vi "arduino -- check responce.vi"(11 "resonse":string) -> (2 "ok?":bool)   [LabVIEW 2020]
uses:
  <vilib>/regexp/Match Regular Expression.xnode
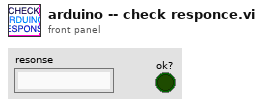
[diagram p1: front panel]
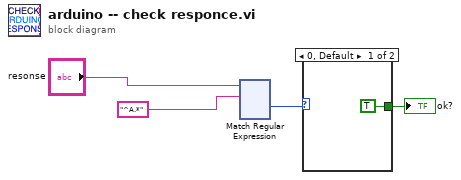
[diagram p0: block diagram]
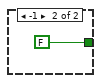
[diagram p2: hidden frame]
diagram:
  n1 = xnode "Match Regular Expression"("input string"="resonse", "regular expression"="^A.*") -> ("offset past match"=w3:i32)  [unwired: 4 in, 4 out]
  n2 = case shown="0, Default" w3 {
    tunnel: [TRUE FALSE] -> w1
    frame 0, Default {
    }
    frame -1 {
    }
  }
  "ok?" <- w1
